vi "VeriStand DSF.Transfer Group.Configuration.Set Section Reference.vi"(10 "Section Ref":T1=18446744073709551615 format="%.0x", 11 "VeriStand DSF.Transfer Group.Configuration in":refnum<class "VeriStand DSF.Transfer Group.Configuration.lvclass">=refnum) -> (3 "VeriStand DSF.Transfer Group.Configuration out":refnum<class "VeriStand DSF.Transfer Group.Configuration.lvclass">)   [LabVIEW 2017, in "Data Sharing Custom Device Engine.lvlib" / "VeriStand DSF.Transfer Group.Configuration.lvclass"]
uses:
  VeriStand DSF.Transfer Group.Configuration.lvclass
  <vilib>/NI Veristand/Custom Device API/Custom Device Item Ref.ctl
  VeriStand DSF.Transfer Group.Configuration.lvclass/VeriStand DSF.Transfer Group.Configuration.ctl
  <vilib>/NI Veristand/Custom Device API/Custom Device API.lvlib
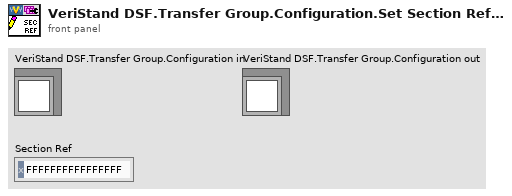
[diagram p1: front panel]
types:
  T1 = typedef "Custom Device API.lvlib/Custom Device Item Ref.ctl" = u64
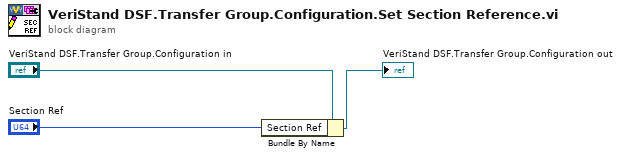
[diagram p0: block diagram]
diagram:
  n1 = Bundle By Name(cluster="VeriStand DSF.Transfer Group.Configuration in", "Section Ref"="Section Ref") -> (→"VeriStand DSF.Transfer Group.Configuration out":refnum<class "VeriStand DSF.Transfer Group.Configuration.lvclass">)
